vi "Strip Trailing Slash.vi"(11 "Path in":string) -> (3 "Path out":string)   [LabVIEW 2020, in "IO.lvlib" / "URI.lvclass"]
uses:
  URI.lvclass
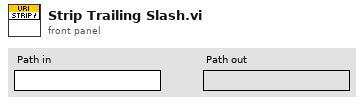
[diagram p1: front panel]
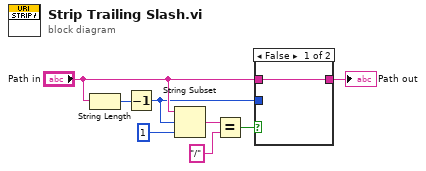
[diagram p0: block diagram]
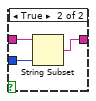
[diagram p2: hidden frame]
diagram:
  n1 = String Length(string="Path in") -> (length=w8:i32)
  n2 = Decrement(x=w8) -> (x-1=w2:i32)
  n3 = String Subset(string="Path in", offset (0)=w2, length (rest)=1 ("length (rest)")) -> (substring=w6:string)
  n4 = Equal?(x=w6, y="/") -> (x = y?=w4:bool)
  n5 = case shown="False" w4 {
    tunnel: "Path in" -> [w9 w12]
    tunnel: w2 -> [_ w11]
    tunnel: [w9 w10] -> w1
    frame False {
    }
    frame True {
      n6 = String Subset(string=w12, length (rest)=w11) -> (substring=w10:string)  [unwired: 1 in]
    }
  }
  "Path out" <- w1
